vi "GetSetGlobalPath2StoreStackData.vi"() -> ()   [LabVIEW 2011]
panel:
  in  "start path":path=path "C:/Entwicklungsdaten/Aktuell/Data"
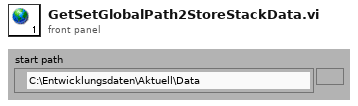
[diagram p1: front panel]
diagram:
